vi "Close Camera mk1.vi"(0 "error out":errorcluster, 1 "IMAQ USB Session Out":T2, 2 "Image":T1) -> ()   [LabVIEW 2011]
uses:
  <vilib>/imaqUSB/imaqUSB.llb/IMAQ USB.ctl
  <vilib>/vision/Image Controls.llb/IMAQ Image.ctl
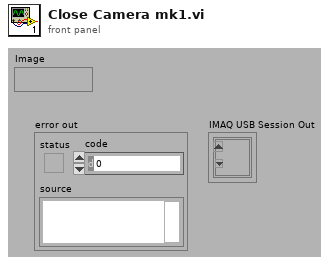
[diagram p1: front panel]
types:
  T1 = typedef "IMAQ Image.ctl" = refnum<image>
  T2 = typedef "IMAQ USB.ctl" = refnum<k1>
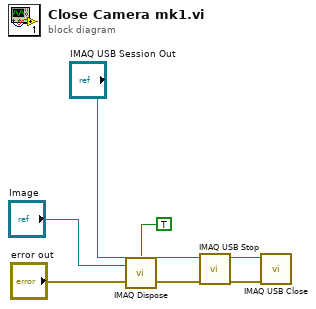
[diagram p0: block diagram]
diagram:
  n1 = call "IMAQ Dispose"("All Images? (No)"=TRUE, "Image"="Image", "error in (no error)"="error out") -> ("error out"=w4:errorcluster)  [unwired: 3 out]
  n2 = call <vilib>:"IMAQ USB Stop.vi"("error in (no error)"=w4, "IMAQ USB Session In"="IMAQ USB Session Out") -> ("error out"=w6:errorcluster, "IMAQ USB Session Out"=w7:T2)  [unwired: 8 out]
  n3 = call <vilib>:"IMAQ USB Close.vi"("error in (no error)"=w6, "IMAQ USB Session In"=w7) -> ()  [unwired: 10 out]
